vi "MeanVariance2D.vi"(0 "3D array":dbl[][][](array[numeric]) format="%.2f") -> (1 "Mean 2D":dbl[][](array[numeric]) format="%.2f", 2 "Standard deviation 2D":dbl[][](array[numeric]) format="%.2f", 3 "Variance 2D":dbl[][](array[numeric]) format="%.2f")   [LabVIEW 2009]
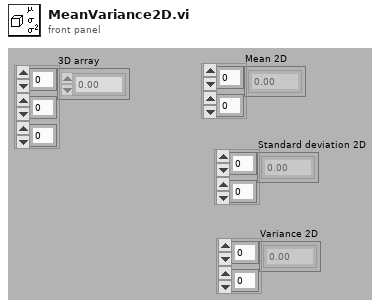
[diagram p1: front panel]
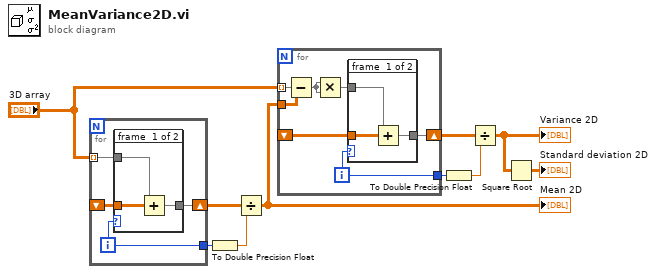
[diagram p0: block diagram]
diagram:
  n1 = for {
    tunnel: "3D array" -> [w12] mode=indexing
    shift-right: [w14] -> w8
    shift-left: _ -> [w13]
    tunnel: [w11] -> w9
    i -> [w11]
    n2 = case shown="1, Default" w11 {
      tunnel: [w17 w18] -> w14
      tunnel: w13 -> [w16 _]
      tunnel: w12 -> [w15 w18]
      frame #0 {
        n3 = Add(x=w15, y=w16) -> (x+y=w17:dbl[][])
      }
      frame #1 {
      }
    }
  }
  n4 = To Double Precision Float(number=w9) -> (double precision float=w10:dbl)
  n5 = Divide(x=w8, y=w10) -> (x/y=w3:dbl[][])
  "Mean 2D" <- w3
  n6 = for {
    tunnel: "3D array" -> [w21] mode=indexing
    shift-right: [w25] -> w7
    shift-left: _ -> [w24]
    tunnel: [w23] -> w6
    tunnel: w3 -> [w22]
    i -> [w23]
    n7 = Subtract(x=w21, y=w22) -> (x-y=w20:dbl[][])
    n8 = Multiply(x=w20, y=w20) -> (x*y=w19:dbl[][])
    n9 = case shown="1, Default" w23 {
      tunnel: [w28 w29] -> w25
      tunnel: w24 -> [w27 _]
      tunnel: w19 -> [w26 w29]
      frame #0 {
        n10 = Add(x=w26, y=w27) -> (x+y=w28:dbl[][])
      }
      frame #1 {
      }
    }
  }
  n11 = To Double Precision Float(number=w6) -> (double precision float=w5:dbl)
  n12 = Divide(x=w7, y=w5) -> (x/y=w2:dbl[][])
  "Variance 2D" <- w2
  n13 = Square Root(x=w2) -> (sqrt(x)=→"Standard deviation 2D":dbl[][])
